vi "Configure Trigger.vi"(7 "Trigger Source (0: Internal)":u16(ring) items=["Internal", "Manual", "External", "Bus"], 8 "error in (no error)":errorcluster, 9 "Step Delay (0.0 sec)":dbl, 10 "Trigger Delay (0.0 sec)":dbl, 11 "VISA resource name":refnum<visa-resource-name>) -> (0 "error out":errorcluster, 3 "VISA resource name out":refnum<visa-resource-name>)   [LabVIEW 2017, in "Agilent E4980.lvlib"]
doc: "Configures the trigger source, the trigger delay and the step delay time."
uses:
  Agilent E4980.lvlib
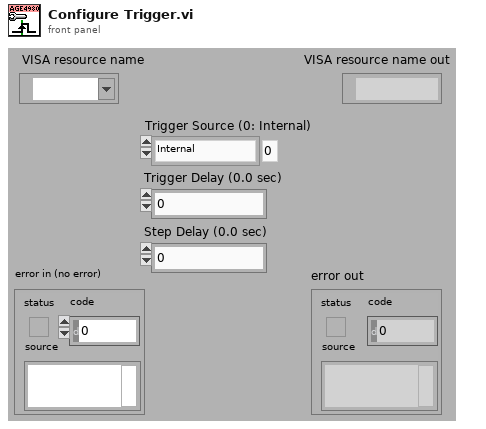
[diagram p1: front panel]
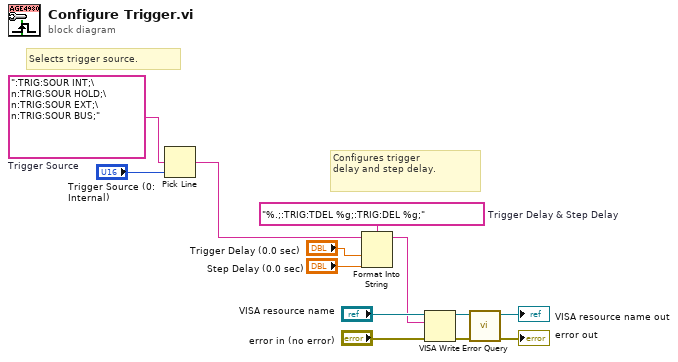
[diagram p0: block diagram]
diagram:
  w5 = "%.;:TRIG:TDEL %g;:TRIG:DEL %g;"  # Trigger Delay & Step Delay
  w10 = ":TRIG:SOUR INT;\n:TRIG:SOUR HOLD;\n:TRIG:SOUR EXT;\n:TRIG:SOUR BUS;"  # Trigger Source
  # "Selects trigger source."
  # "Configures trigger\ndelay and step delay."
  n1 = Pick Line(multi-line string=w10, line index="Trigger Source (0: Internal)") -> (output string=w2:string)  [unwired: 1 in]
  n2 = Format Into String(format string=w5, initial string=w2, "Trigger Delay (0.0 sec)", "Step Delay (0.0 sec)") -> (resulting string=w1:string)  [unwired: 1 in, 1 out]
  n3 = VISA Write(VISA resource name="VISA resource name", write buffer=w1, error in (no error)="error in (no error)") -> (VISA resource name out=w7:refnum<visa-resource-name>, error out=w6:errorcluster)  [unwired: 1 out]
  n4 = call "Error Query.vi"("error in (no error)"=w6, "VISA resource name"=w7) -> ("error out"=→"error out":errorcluster, "VISA resource name out"=→"VISA resource name out":refnum<visa-resource-name>)  [unwired: 6 in, 2 out]
